vi "Get Head Model.vi"(8 "error in (no error)":errorcluster, 11 "name":string) -> (0 "error out":errorcluster, 2 "function return":u32, 3 "name out":string)   [LabVIEW 2014, in "atmcd32d.lvlib"]
doc: "unsigned int WINAPI GetHeadModel(char * name);"
uses:
  atmcd32d.lvlib
  atmcd32d.dll
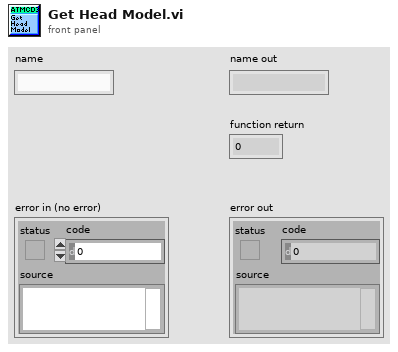
[diagram p1: front panel]
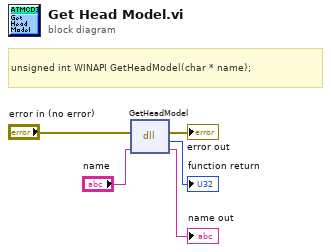
[diagram p0: block diagram]
diagram:
  # "unsigned int WINAPI GetHeadModel(char * name);"
  n1 = dll-call lib="C:/Users/Bakir/Documents/Lambda2-Testing/lib/Andorlib/atmcd32d.*" fn="GetHeadModel"(error in="error in (no error)", "name"="name") -> (error out=→"error out":errorcluster, →"function return":u32, "name"=→"name out":string)  [unwired: 2 in, 1 out]
